vi "MetaClientQueueTCP.vi"(8 "error in (no error)":errorcluster, 10 "Enum":enum16{"shutdown", "send_queue", "get_queue"}(ring), 11 "RefIn":refnum<vi>) -> (0 "error out":errorcluster, 3 "RefOut":refnum<vi>)   [LabVIEW 2019]
uses:
  QueueControl.ctl
panel:
  # "Queue :"
  # "Queue :"
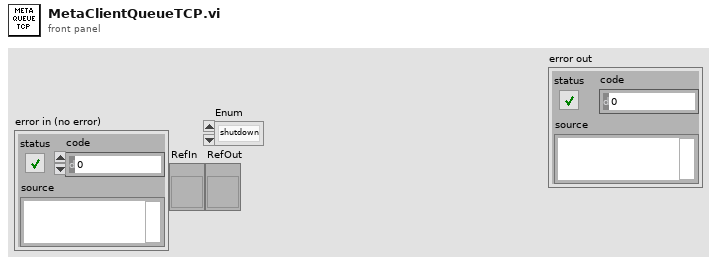
[diagram p1: front panel]
types:
  T1 = enum16{"Standard", "Buffered", "CRLF", "Immediate"}
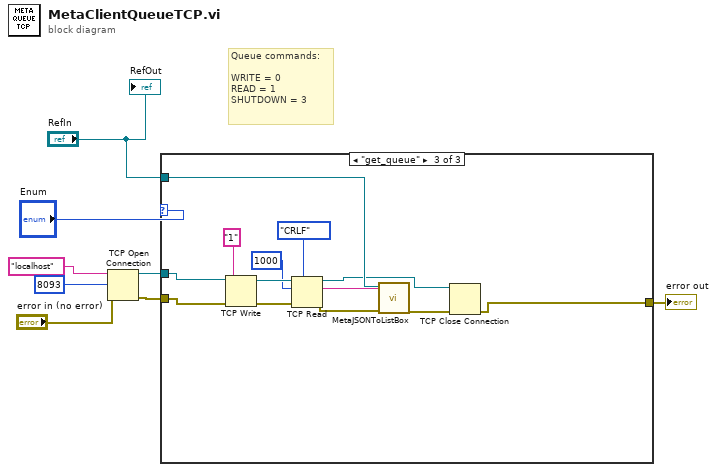
[diagram p0: block diagram]
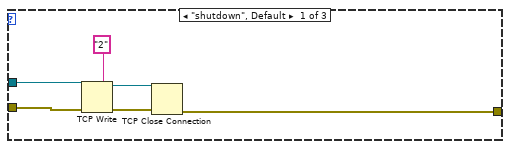
[diagram p2: hidden frame]
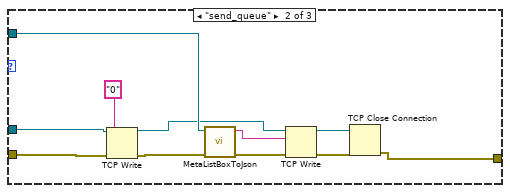
[diagram p3: hidden frame]
diagram:
  # "Queue commands:\n\nWRITE = 0\nREAD = 1\nSHUTDOWN = 3"
  n1 = TCP Open Connection(address="localhost", remote port or service name=u16 8093, error in (no error)="error in (no error)") -> (connection ID=w5:refnum<k5>, error out=w4:errorcluster)  [unwired: 2 in]
  n2 = case shown="\"get_queue\"" "Enum" {
    tunnel: w5 -> [w12 w25 w36]
    tunnel: w4 -> [w13 w24 w37]
    tunnel: "RefIn" -> [_ w20 w28]
    tunnel: [w9 w15 w26] -> w2
    frame "shutdown", Default {
      n3 = TCP Write(connection ID=w12, data in="2", error in (no error)=w13) -> (connection ID out=w11:refnum<k5>, error out=w10:errorcluster)  [unwired: 1 in, 1 out]
      n4 = TCP Close Connection(connection ID=w11, error in (no error)=w10) -> (error out=w9:errorcluster)  [unwired: 1 in, 1 out]
    }
    frame "send_queue" {
      n5 = TCP Write(connection ID=w25, data in="0", error in (no error)=w24) -> (connection ID out=w18:refnum<k5>, error out=w22:errorcluster)  [unwired: 1 in, 1 out]
      n6 = call "MetaListBoxToJson.vi"("error in (no error)"=w22, "ref in 2"=w20) -> ("error out"=w21:errorcluster, "JSON queue ou"=w19:string)  [unwired: 8 in]
      n7 = TCP Write(connection ID=w18, data in=w19, error in (no error)=w21) -> (connection ID out=w17:refnum<k5>, error out=w16:errorcluster)  [unwired: 1 in, 1 out]
      n8 = TCP Close Connection(connection ID=w17, error in (no error)=w16) -> (error out=w15:errorcluster)  [unwired: 1 in, 1 out]
    }
    frame "get_queue" {
      n9 = TCP Write(connection ID=w36, data in="1", error in (no error)=w37) -> (connection ID out=w35:refnum<k5>, error out=w34:errorcluster)  [unwired: 1 in, 1 out]
      n10 = TCP Read(connection ID=w35, bytes to read=1000, error in (no error)=w34, 7:T1."CRLF" ("mode (standard)")) -> (connection ID out=w27:refnum<k5>, data out=w29:string, error out=w30:errorcluster)  [unwired: 1 in]
      n11 = call "MetaJSONToListBox.vi"("error in (no error)"=w30, "JSON queue in"=w29, "RefIn"=w28) -> ("error out"=w31:errorcluster)  [unwired: 8 in]
      n12 = TCP Close Connection(connection ID=w27, error in (no error)=w31) -> (error out=w26:errorcluster)  [unwired: 1 in, 1 out]
    }
  }
  "error out" <- w2
  "RefOut" <- "RefIn"
